vi "Calculate Samples.vi"(8 "error in (no error)":errorcluster, 11 "Sine Stimulus in":refnum<class "Sine Stimulus.lvclass">) -> (0 "error out":errorcluster, 3 "Sine Stimulus out":refnum<class "Sine Stimulus.lvclass">)   [LabVIEW 2015, in "Sine Stimulus.lvclass"]
uses:
  Sine Stimulus.lvclass
  Sine Stimulus.lvclass/Sine Stimulus.ctl
  <vilib>/Analysis/NI_AALBase.lvlib
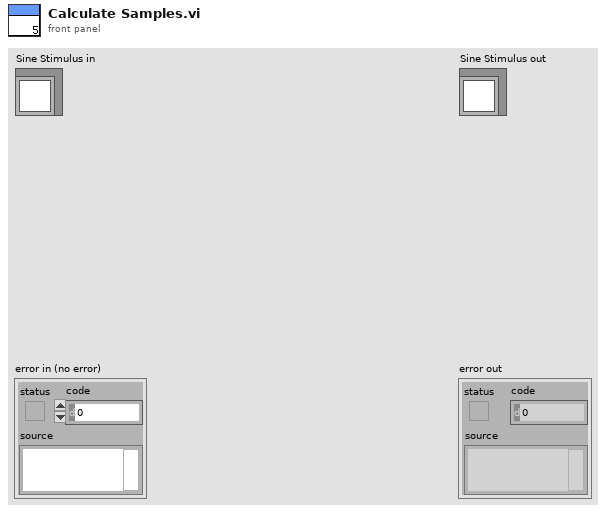
[diagram p1: front panel]
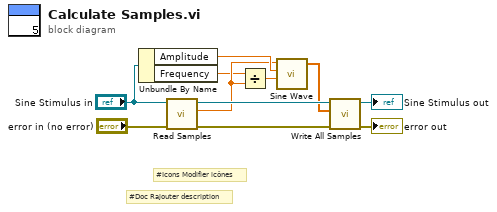
[diagram p0: block diagram]
diagram:
  # "#Doc Rajouter description"
  # "#Icons Modifier icônes"
  n1 = Unbundle By Name("Sine Stimulus in") -> ("Amplitude"=w9:dbl, "Frequency"=w1:dbl)
  n2 = call-dynamic "Read Samples.vi"("error in (no error)"="error in (no error)", "Stimulus in"="Sine Stimulus in") -> ("error out"=w3:errorcluster, "Samples"=w8:dbl, "Stimulus out"=w11:refnum<class "Sine Stimulus.lvclass">)  [unwired: 7 in]
  n3 = Divide(x=w1, y=w8) -> (x/y=w7:dbl)
  n4 = call <vilib>:"Sine Wave.vi"("samples"=w8, "amplitude"=w9, "frequency"=w7) -> ("sine wave"=w6:dbl[])  [unwired: 2 in, 2 out]
  n5 = call-dynamic "Write All Samples.vi"("error in (no error)"=w3, "All Samples"=w6, "Stimulus in"=w11) -> ("error out"=→"error out":errorcluster, "Stimulus out"=→"Sine Stimulus out":refnum<class "Sine Stimulus.lvclass">)  [unwired: 7 in]
